vi "Log.vi"(8 "error in (no error)":errorcluster, 10 "LogRecord":refnum<class "LogRecord.lvclass">, 11 "EventLogHandle in":refnum<class "EventLogHandle.lvclass">) -> (0 "error out":errorcluster, 3 "EventLogHandle out":refnum<class "EventLogHandle.lvclass">)   [LabVIEW 2024, in "EventLogHandle.lvclass"]
uses:
  EventLogHandle.lvclass
  Record/LogRecord.lvclass
  EventLogHandle.lvclass/EventLogHandle.ctl
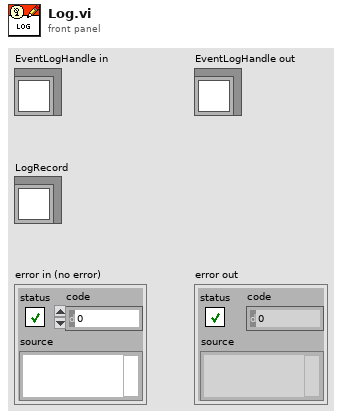
[diagram p1: front panel]
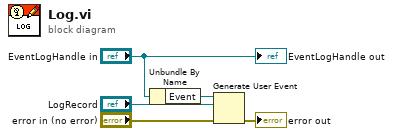
[diagram p0: block diagram]
diagram:
  n1 = Unbundle By Name("EventLogHandle in") -> ("Event"=w4:refnum<user-event>)
  n2 = Generate User Event(user event=w4, event data cluster="LogRecord", error in="error in (no error)") -> (error out=→"error out":errorcluster)  [unwired: 1 in, 1 out]
  "EventLogHandle out" <- "EventLogHandle in"
